vi "Get Control Information.vi"(8 "error in (no error)":errorcluster, 11 "Listbox in":refnum<class "Listbox.lvclass">) -> (0 "error out":errorcluster, 2 "Control Information":string[][](array[string]), 3 "Listbox out":refnum<class "Listbox.lvclass">)   [LabVIEW 2017, in "Localization.lvlib" / "Listbox.lvclass"]
doc: "VI for override that is supposed to do go throgh the process for each control type and pull out the information that is necessary for each control.\n\nChoose Movement Consulting, LLC"
uses:
  Listbox.lvclass
  C:/Apps/CMC/OpenSource/Localization/Control Info/Control Info.lvclass
  Localization.lvlib
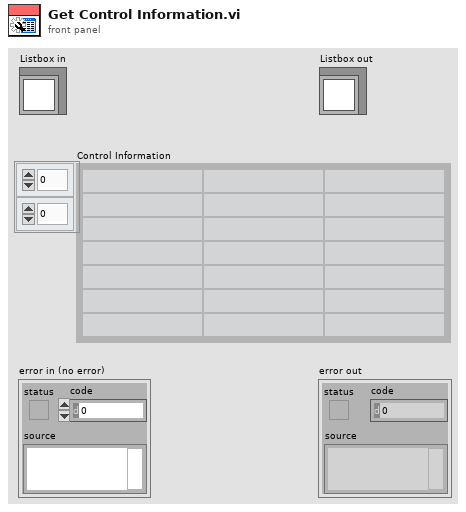
[diagram p1: front panel]
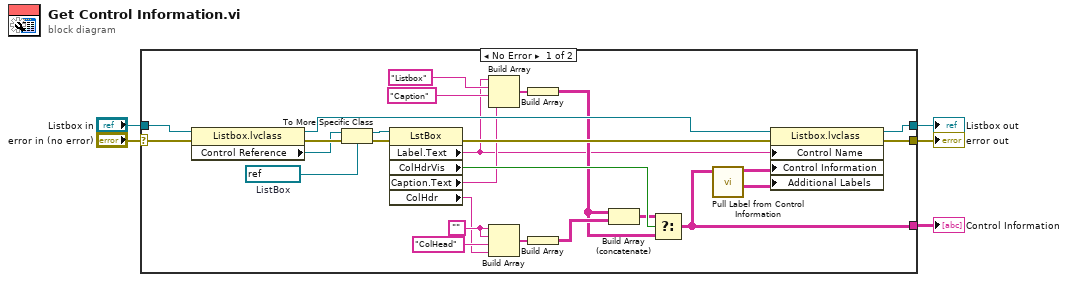
[diagram p0: block diagram]
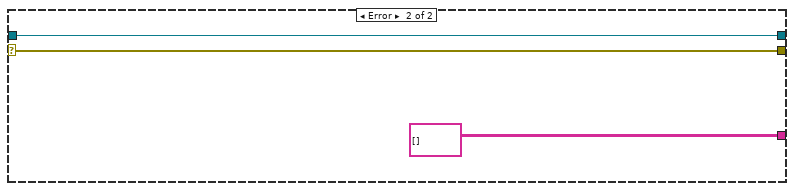
[diagram p2: hidden frame]
diagram:
  n1 = case shown="No Error" "error in (no error)" {
    selector: "error in (no error)" -> [w27 w35]
    tunnel: [w23 w35] -> w2
    tunnel: "Listbox in" -> [w26 w34]
    tunnel: [w9 string[][] []] -> w3
    tunnel: [w21 w34] -> w1
    frame No Error {
      w12 = ""
      w32 = refnum<vi> refnum  # ListBox
      n2 = property class="Listbox.lvclass"(reference=w26, error in=w27) -> (reference out=w22:refnum<class "Listbox.lvclass">, error out=w28:errorcluster, "Control Reference"=w25:refnum<vi>)
      n3 = To More Specific Class(target class=w32, reference=w25, error in=w28) -> (specific class reference=w31:refnum<vi>, error out=w29:errorcluster)
      n4 = property class="LstBox"(reference=w31, error in=w29) -> (error out=w24:errorcluster, "Label.Text"=w6:string, "ColHdrVis"=w20:bool, "Caption.Text"=w11:string, "ColHdr"=w10:string)  [unwired: 1 out]
      n5 = Build Array(w6, "Listbox", "Caption", w11) -> (w30:string[])
      n6 = Build Array(w12, w12, "ColHead", w10) -> (w13:string[])
      n7 = Build Array(w30) -> (w17:string[][])
      n8 = Build Array(w13) -> (w18:string[][])
      n9 = Build Array (concatenate)(w17, w18) -> (w16:string[][])
      n10 = Select(t=w16, s=w20, f=w17) -> (s? t:f=w9:string[][])
      n11 = call "Pull Label from Control Information.vi"("Control Caption Table"=w9) -> ("Additional Labels"=w7:string[][], "Control Information"=w8:string[][])  [unwired: 9 in]
      n12 = property class="Listbox.lvclass"(reference=w22, error in=w24, "Control Name"=w6, "Control Information"=w8, "Additional Labels"=w7) -> (reference out=w21:refnum<class "Listbox.lvclass">, error out=w23:errorcluster)
    }
    frame Error {
    }
  }
  "error out" <- w2
  "Listbox out" <- w1
  "Control Information" <- w3
